vi "Pre Launch Init.vi"(11 "Mediator in":refnum<class "Mediator.lvclass">) -> (0 "error out":errorcluster, 3 "Mediator out":refnum<class "Mediator.lvclass">)   [LabVIEW 2015, in "Mediator.lvlib" / "Mediator.lvclass"]
doc: "(<B>Filename</B>: Actor Framework.lvlib:Actor.lvclass:Pre Launch Init.vi)\n\nDefines behavior that occurs after the Launch Nested Actor method is invoked but before the actor's Actor Core method begins running.\n\nBy default, this method does nothing. A descendant class may override it to define behavior."
uses:
  Mediator.lvclass
  Mediator.lvclass/Mediator.ctl
  IMediator/IMediator/IMediator.lvclass
  TopicLookupTable/TopicLookupTable.lvclass
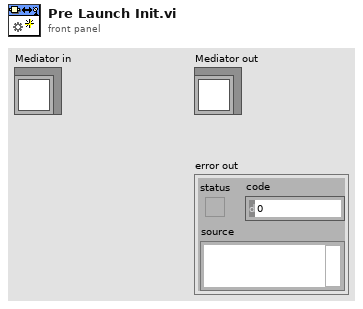
[diagram p1: front panel]
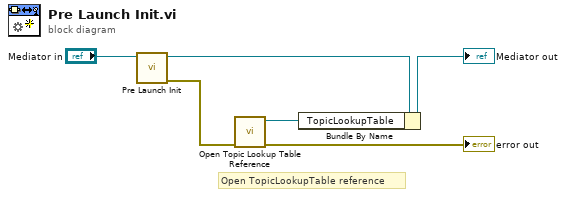
[diagram p0: block diagram]
diagram:
  # "Open TopicLookupTable reference"
  n1 = call-parent "Pre Launch Init.vi"("Actor in"="Mediator in") -> ("error out"=w2:errorcluster, "Actor out"=w6:refnum<class "Mediator.lvclass">)  [unwired: 9 in]
  n2 = call "Open Topic Lookup Table Reference.vi"("error in (no error)"=w2) -> ("error out"=→"error out":errorcluster, "TopicLookupTable Reference"=w3:refnum<data-value>)  [unwired: 9 in]
  n3 = Bundle By Name(cluster=w6, "TopicLookupTable"=w3) -> (→"Mediator out":refnum<class "Mediator.lvclass">)
